vi "Base64_Decode CORE.vi"(1 "Decode LUT":u32[](array[numeric]), 2 "Base64 String":string) -> (0 "string":string)   [LabVIEW 2017, in "Serializer.Base64.lvclass"]
doc: "20250509 - CORE function created to allow LUT variable input support of fast Base64url decoding"
uses:
  Serializer.Base64.lvclass
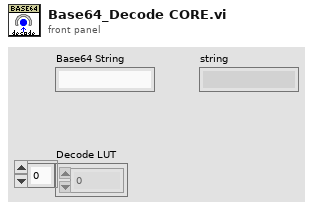
[diagram p1: front panel]
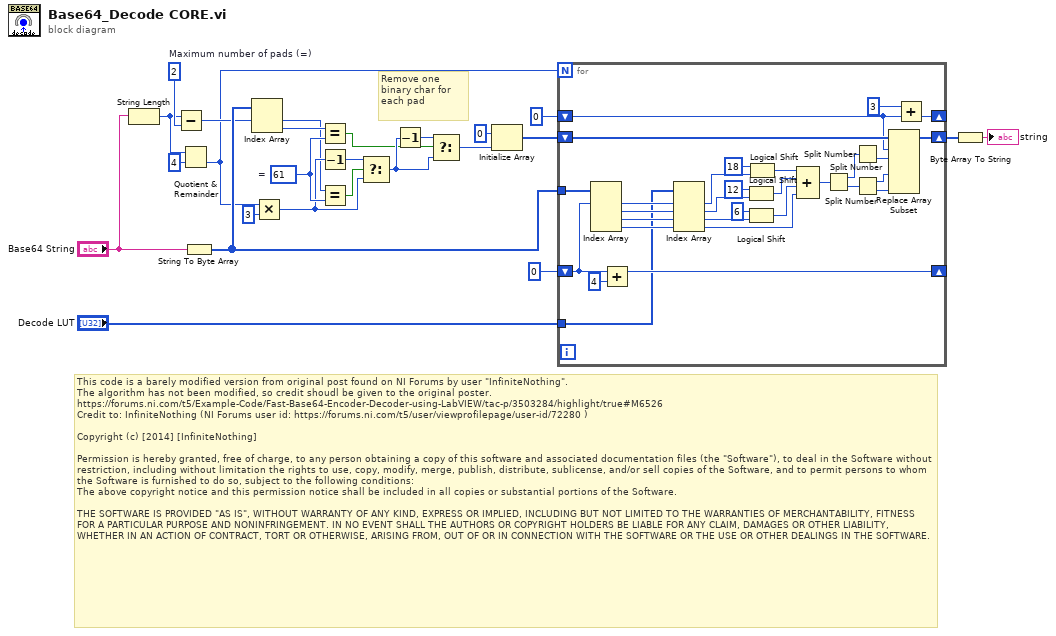
[diagram p0: block diagram]
diagram:
  w23 = u8 61  # =
  w9 = 2  # Maximum number of pads (=)
  # "This code is a barely modified version from original post found on NI Forums by user \"InfiniteNothing\".\nThe algorithm has not been modified, so credit shoudl be given to the original poster.\nhttps://forums.ni.com/t5/Example-Code/Fast-Base64-Encoder-Decoder-using-LabVIEW/tac-p/3503284/highlight/true#M6526\nCredit to: InfiniteNothing (NI Forums user id: https://forums.ni.com/t5/user/viewprofilepage/user-id/72280 )\n\nCopyright (c) [2014] [InfiniteNothing]\n\nPermission is hereby granted, free of charge, to any person obtaining a copy of this software and associated documentation files (the \"Software\"), to deal in the Software without restriction, including without limitation the rights to use, copy, modify, merge, publish, distribute, sublicense, and/or sell copies of the Software, and to permit persons to whom the Software is furnished to do so, subject to the following conditions:\nThe above copyright notice and this permission notice shall be included in all copies or substantial portions of the Software.\n\nTHE SOFTWARE IS PROVIDED \"AS IS\", WITHOUT WARRANTY OF ANY KIND, EXPRESS OR IMPLIED, INCLUDING BUT NOT LIMITED TO THE WARRANTIES OF MERCHANTABILITY, FITNESS FOR A PARTICULAR PURPOSE AND NONINFRINGEMENT. IN NO EVENT SHALL THE AUTHORS OR COPYRIGHT HOLDERS BE LIABLE FOR ANY CLAIM, DAMAGES OR OTHER LIABILITY, WHETHER IN AN ACTION OF CONTRACT, TORT OR OTHERWISE, ARISING FROM, OUT OF OR IN CONNECTION WITH THE SOFTWARE OR THE USE OR OTHER DEALINGS IN THE SOFTWARE."
  # "Remove one binary char for each pad"
  n1 = String Length(string="Base64 String") -> (length=w8:i32)
  n2 = Subtract(x=w8, y=w9) -> (x-y=w10:i32)
  n3 = Quotient & Remainder(x=w8, y=4 ("U64 Chars")) -> (floor(x/y)=w4:i32)  [unwired: 1 out]
  n4 = String To Byte Array(string="Base64 String") -> (unsigned byte array=w25:u8[])
  n5 = Index Array(array=w25, index #1=w10) -> (element #1=w11:u8, element #2=w12:u8)  [unwired: 1 in]
  n6 = Multiply(x=w4, y=3 ("Binary chars")) -> (x*y=w18:i32)
  n7 = Equal?(x=w12, y=w23) -> (x = y?=w16:bool)
  n8 = Decrement(x=w18) -> (x-1=w17:i32)
  n9 = Equal?(x=w11, y=w23) -> (x = y?=w14:bool)
  n10 = Select(t=w17, s=w14, f=w18) -> (s? t:f=w19:i32)
  n11 = Decrement(x=w19) -> (x-1=w20:i32)
  n12 = Select(t=w20, s=w16, f=w19) -> (s? t:f=w15:i32)
  n13 = Initialize Array(u8 0 ("element"), w15) -> (w1:u8[])
  n14 = for {
    N: w4 -> [_]
    tunnel: w25 -> [w50]
    shift-right: [w48] -> _
    shift-left: 0 ("B64 Index") -> [w49]
    shift-right: [w44] -> _
    shift-left: 0 ("Binary Index") -> [w43]
    shift-right: [w46] -> w13
    shift-left: w1 -> [w47]
    tunnel: "Decode LUT" -> [w26]
    n15 = Index Array(array=w50, index #1=w49) -> (element #1=w34:u8, element #2=w33:u8, element #3=w32:u8, element #4=w31:u8)  [unwired: 3 in]
    n16 = Add(x=w49, y=4 ("B64s per 3 U8s")) -> (x+y=w48:i32)
    n17 = Index Array(array=w26, index #1=w34, index #2=w33, index #3=w32, index #4=w31) -> (element #1=w30:u32, element #2=w29:u32, element #3=w28:u32, element #4=w27:u32)
    n18 = Logical Shift(y=12, x=w29) -> (x << y=w37:u32)
    n19 = Logical Shift(y=6, x=w28) -> (x << y=w36:u32)
    n20 = Logical Shift(y=18, x=w30) -> (x << y=w38:u32)
    n21 = Compound Arithmetic op=ADD(w38, w37, w36, w27) -> (w35:u32)
    n22 = Split Number(x=w35) -> (hi(x)=w54:u16, lo(x)=w55:u16)
    n23 = Split Number(x=w54) -> (lo(x)=w53:u8)  [unwired: 1 out]
    n24 = Split Number(x=w55) -> (hi(x)=w52:u8, lo(x)=w51:u8)
    n25 = Replace Array Subset(array=w47, new element #1=w53, index #1=w43, new element #2=w52, new element #3=w51) -> (w46:u8[])  [unwired: 2 in]
    n26 = Add(x=3 ("Binary Chars per 4 B64s"), y=w43) -> (x+y=w44:i32)
  }
  n27 = Byte Array To String(unsigned byte array=w13) -> (string=→"string":string)
